vi "CV_measure_LCR.vi"(0 "Input parameters":T2={"Measurement type"=enum."Debug", "Sensor type"=enum."HPK_8in_256", "Identifier"="test.txt", "Open after execution?"=FALSE, "Plot after execution?"=FALSE, "Display channel"=0, "Voltage Delay (s)"=0.5, "Switch Delay (s)"=0.01, "VISA resource name source"="", "VISA resource name DMM"="", "VISA resource name LCR"="", "Compliance  Level (A)"=10.0, "Voltage Limit (V)"=1000.0, "Data storage location"="", "Scan voltages"="", "Use source as DMM?"=FALSE, "LCR signal frequenzy (Hz)"=10.0, "DMM device"=enum."Keithley2001", "Sampling number"=1, "Use env. sensors on"=enum."Sensirion sht1x/7x", "Switchboard Handle"=0, "Use Switchboard"=FALSE, "LCR signal voltage (V)"=10000.0, "Repeat"=1, "Scan voltages IV"="", "Scan voltages CV"="", "Hex pad numbers?"=FALSE, "Set measurement type"=enum."Debug", "Custom pad scan"="", "IV voltage Delay (s)"=0.5, "CV voltage Delay (s)"=0.5, "Needle measurement?"=FALSE, "Comments"="test.txt", "LCR signal frequenzy (kHz)"=10.0, "Compliance  Level (uA)"=10.0, "Open Correction Array"=array2304x3[6912 elements], "Current set voltage"=0.0, "Last set voltage"=0.0, "Current channel"=0, "Last OpenCorrection index"=-1, "Total curr/vltg every x steps"=10, "Current channel iteration"=0, "No CV corrections"=FALSE, "Mapfile"="", "Corrfile"="", "Invert polarity"=FALSE, "IV voltage file"=path "", "CV voltage file"=path "", "IV Switch Delay (s)"=0.01, "CV Switch Delay (s)"=0.01} {"CV Switch Delay (s)" format="%#_13g"; "IV Switch Delay (s)" format="%#_13g"; "Last set voltage" format="%#_13g"; "Current set voltage" format="%#_13g"; "CV voltage Delay (s)" format="%#_13g"; "IV voltage Delay (s)" format="%#_13g"; "Voltage Limit (V)" format="%#_13g"; "Voltage Delay (s)" format="%#_13g"; "Switch Delay (s)" format="%#_13g"}, 11 "error in (no error)":errorcluster) -> (4 "Input parameters out":T2={"Measurement type"=enum."Debug", "Sensor type"=enum."HPK_8in_256", "Identifier"="test.txt", "Open after execution?"=FALSE, "Plot after execution?"=FALSE, "Display channel"=0, "Voltage Delay (s)"=0.5, "Switch Delay (s)"=0.01, "VISA resource name source"="", "VISA resource name DMM"="", "VISA resource name LCR"="", "Compliance  Level (A)"=10.0, "Voltage Limit (V)"=1000.0, "Data storage location"="", "Scan voltages"="", "Use source as DMM?"=FALSE, "LCR signal frequenzy (Hz)"=10.0, "DMM device"=enum."Keithley2001", "Sampling number"=1, "Use env. sensors on"=enum."Sensirion sht1x/7x", "Switchboard Handle"=0, "Use Switchboard"=FALSE, "LCR signal voltage (V)"=10000.0, "Repeat"=1, "Scan voltages IV"="", "Scan voltages CV"="", "Hex pad numbers?"=FALSE, "Set measurement type"=enum."Debug", "Custom pad scan"="", "IV voltage Delay (s)"=0.5, "CV voltage Delay (s)"=0.5, "Needle measurement?"=FALSE, "Comments"="test.txt", "LCR signal frequenzy (kHz)"=10.0, "Compliance  Level (uA)"=10.0, "Open Correction Array"=array2304x3[6912 elements], "Current set voltage"=0.0, "Last set voltage"=0.0, "Current channel"=0, "Last OpenCorrection index"=-1, "Total curr/vltg every x steps"=10, "Current channel iteration"=0, "No CV corrections"=FALSE, "Mapfile"="", "Corrfile"="", "Invert polarity"=FALSE, "IV voltage file"=path "", "CV voltage file"=path "", "IV Switch Delay (s)"=0.01, "CV Switch Delay (s)"=0.01} {"CV Switch Delay (s)" format="%#_13g"; "IV Switch Delay (s)" format="%#_13g"; "Last set voltage" format="%#_13g"; "Current set voltage" format="%#_13g"; "CV voltage Delay (s)" format="%#_13g"; "IV voltage Delay (s)" format="%#_13g"; "Voltage Limit (V)" format="%#_13g"; "Voltage Delay (s)" format="%#_13g"; "Switch Delay (s)" format="%#_13g"}, 8 "LCR data":T1, 15 "error out":errorcluster)   [LabVIEW 2016]
uses:
  input_params.ctl
  data_LCR.ctl
  <instrlib>/Agilent E4980/Agilent E4980.lvlib
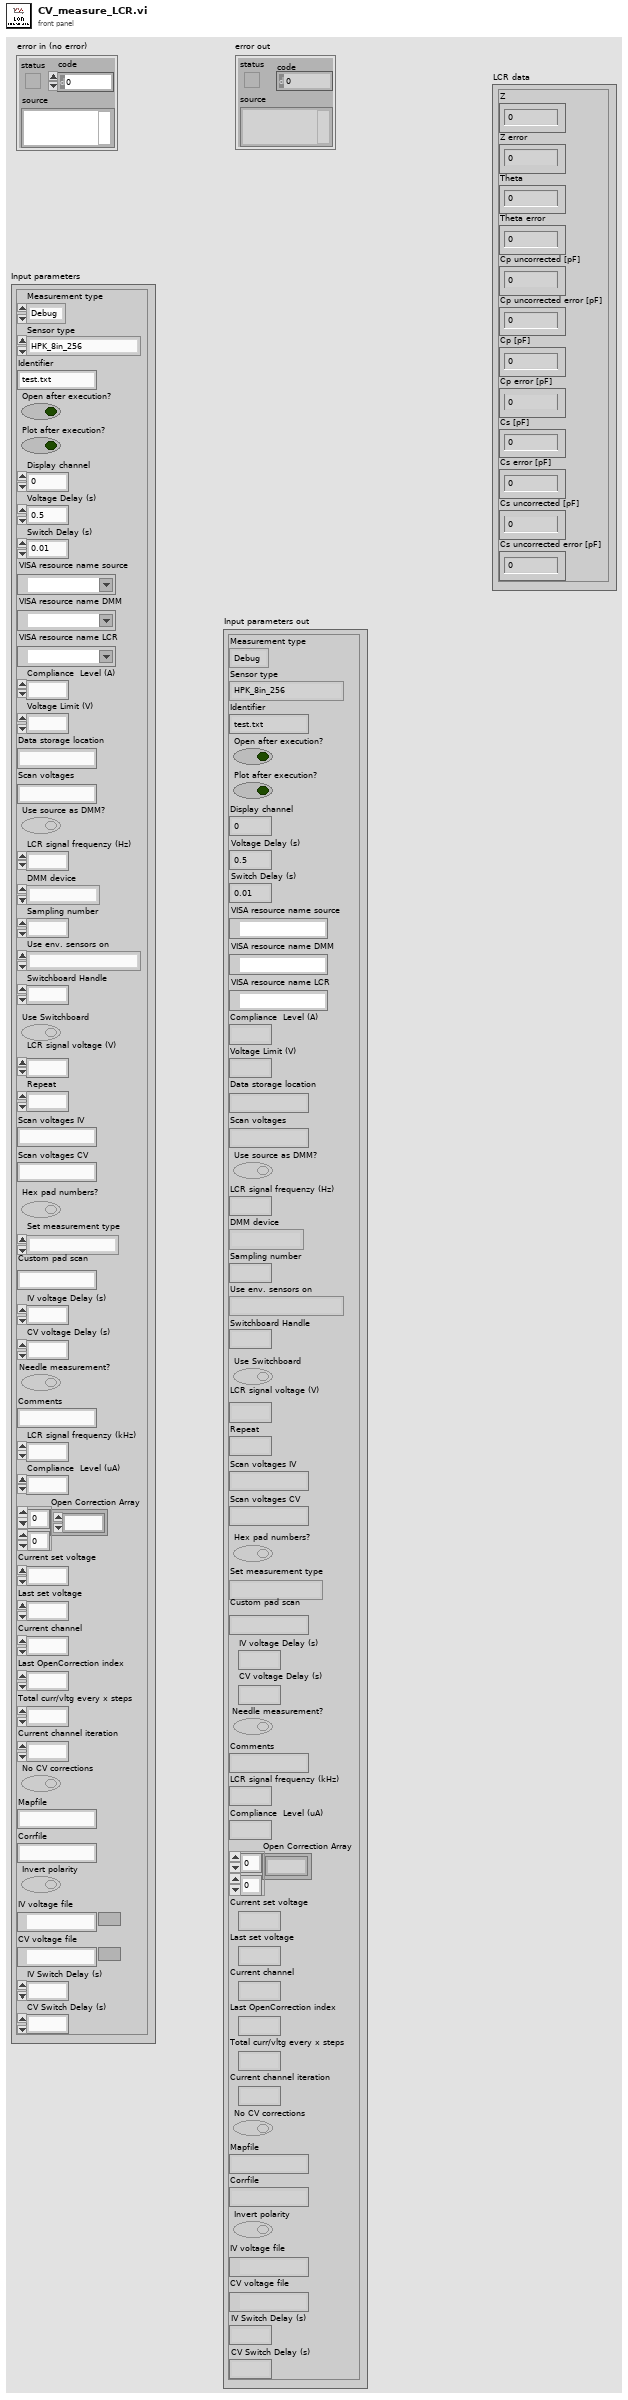
[diagram p1: front panel]
types:
  T1 = typedef "data_LCR.ctl" = cluster{"Z":dbl, "Z error":dbl, "Theta":dbl, "Theta error":dbl, "Cp uncorrected [pF]":dbl, "Cp uncorrected error [pF]":dbl, "Cp [pF]":dbl, "Cp error [pF]":dbl, "Cs [pF]":dbl, "Cs error [pF]":dbl, "Cs uncorrected [pF]":dbl, "Cs uncorrected error [pF]":dbl}
  T2 = typedef "input_params.ctl" = cluster{"Measurement type":enum16{"IV", "CV", "Debug", "Test_contact"}, "Sensor type":enum16{"HPK_6in_135", "HPK_8in_256", "IFX_8in_256", "Diode", "HPK_6in_256", "Full matrix"}, "Identifier":string, "Open after execution?":bool, "Plot after execution?":bool, "Display channel":i32, "Voltage Delay (s)":dbl, "Switch Delay (s)":dbl, "VISA resource name source":refnum<visa-resource-name>, "VISA resource name DMM":refnum<visa-resource-name>, "VISA resource name LCR":refnum<visa-resource-name>, "Compliance  Level (A)":dbl, "Voltage Limit (V)":dbl, "Data storage location":string, "Scan voltages":string, "Use source as DMM?":bool, "LCR signal frequenzy (Hz)":dbl, "DMM device":enum16{"Keithley2001", "Keithley2450", "Keithley2410", "Keithley6487"}, "Sampling number":i32, "Use env. sensors on":enum16{"Sensirion sht1x/7x", "Switch Matrix", "Probecard"}, "Switchboard Handle":u32, "Use Switchboard":bool, "LCR signal voltage (V)":dbl, "Repeat":i32, "Scan voltages IV":string, "Scan voltages CV":string, "Hex pad numbers?":bool, "Set measurement type":enum16{"IV", "CV", "Debug", "Test_contact", "IV+CV"}, "Custom pad scan":string, "IV voltage Delay (s)":dbl, "CV voltage Delay (s)":dbl, "Needle measurement?":bool, "Comments":string, "LCR signal frequenzy (kHz)":dbl, "Compliance  Level (uA)":dbl, "Open Correction Array":dbl[][], "Current set voltage":dbl, "Last set voltage":dbl, "Current channel":i32, "Last OpenCorrection index":i32, "Total curr/vltg every x steps":i32, "Current channel iteration":i32, "No CV corrections":bool, "Mapfile":string, "Corrfile":string, "Invert polarity":bool, "IV voltage file":path, "CV voltage file":path, "IV Switch Delay (s)":dbl, "CV Switch Delay (s)":dbl}
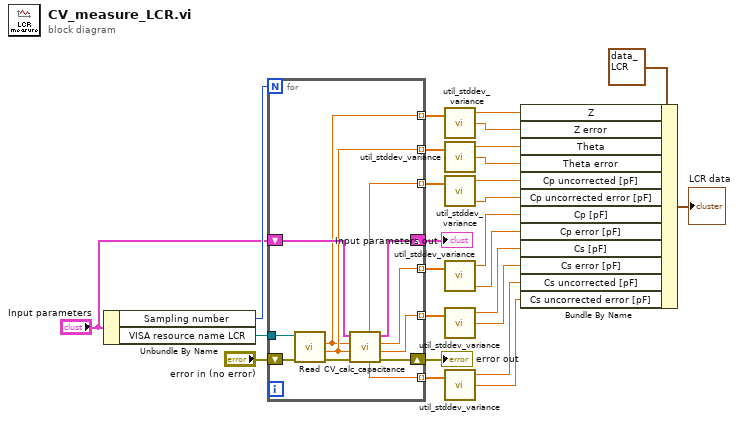
[diagram p0: block diagram]
diagram:
  n1 = Unbundle By Name("Input parameters") -> ("Sampling number"=w23:i32, "VISA resource name LCR"=w25:refnum<visa-resource-name>)
  n2 = for {
    N: w23 -> [_]
    tunnel: w25 -> [w38]
    tunnel: [w30] -> w20 mode=indexing
    tunnel: [w29] -> w19 mode=indexing
    tunnel: [w31] -> w22 mode=indexing
    tunnel: [w32] -> w21 mode=indexing
    shift-right: [w35] -> w26
    shift-left: "error in (no error)" -> [w37]
    tunnel: [w28] -> w16 mode=indexing
    tunnel: [w27] -> w15 mode=indexing
    shift-right: [w33] -> w17
    shift-left: "Input parameters" -> [w34]
    n3 = call <instrlib>:"Read.vi"("error in (no error)"=w37, "VISA resource name"=w38) -> ("error out"=w36:errorcluster, "Secondary Parameter"=w32:dbl, "Primary Parameter"=w31:dbl)  [unwired: 6 in, 1 out]
    n4 = call "CV_calc_capacitance.vi"("error in (no error)"=w36, "Theta (Phase)"=w32, "Z (impedance)"=w31, "Input parameters"=w34) -> ("error out"=w35:errorcluster, "Cs [pF]"=w29:dbl, "Cp [pF]"=w30:dbl, "Input parameters out"=w33:T2, "Cs uncorrected [pF]"=w27:dbl, "Cp uncorrected [pF]"=w28:dbl)  [unwired: 2 in]
  }
  "error out" <- w26
  "Input parameters out" <- w17
  n5 = call "util_stddev_variance.vi"("X"=w22) -> ("mean"=w2:dbl, "standard deviation"=w3:dbl)  [unwired: 1 in, 1 out]
  n6 = call "util_stddev_variance.vi"("X"=w21) -> ("mean"=w1:dbl, "standard deviation"=w4:dbl)  [unwired: 1 in, 1 out]
  n7 = call "util_stddev_variance.vi"("X"=w16) -> ("mean"=w5:dbl, "variance"=w6:dbl)  [unwired: 1 in, 1 out]
  n8 = call "util_stddev_variance.vi"("X"=w20) -> ("mean"=w7:dbl, "variance"=w8:dbl)  [unwired: 1 in, 1 out]
  n9 = call "util_stddev_variance.vi"("X"=w19) -> ("mean"=w9:dbl, "standard deviation"=w10:dbl)  [unwired: 1 in, 1 out]
  n10 = call "util_stddev_variance.vi"("X"=w15) -> ("mean"=w11:dbl, "standard deviation"=w12:dbl)  [unwired: 1 in, 1 out]
  n11 = Bundle By Name(cluster=T1 {"Z"=0.0, "Z error"=0.0, "Theta"=0.0, "Theta error"=0.0, "Cp uncorrected [pF]"=0.0, "Cp uncorrected error [pF]"=0.0, "Cp [pF]"=0.0, "Cp error [pF]"=0.0, "Cs [pF]"=0.0, "Cs error [pF]"=0.0, "Cs uncorrected [pF]"=0.0, "Cs uncorrected error [pF]"=0.0} ("Cluster"), "Z"=w2, "Z error"=w3, "Theta"=w1, "Theta error"=w4, "Cp uncorrected [pF]"=w5, "Cp uncorrected error [pF]"=w6, "Cp [pF]"=w7, "Cp error [pF]"=w8, "Cs [pF]"=w9, "Cs error [pF]"=w10, "Cs uncorrected [pF]"=w11, "Cs uncorrected error [pF]"=w12) -> (→"LCR data":T1)
